vi "new_cursor.vi"(10 "XY":cluster{"X":dbl, "Y":dbl}, 11 "CrsrList":T1(array[cluster])) -> (3 "CrsrList Out":T1(array[cluster]))   [LabVIEW 2023]
panel:
  out "output array":string[](array[string])
  out "Array":bool[](array[boolean])
  out "s? t:f":i32
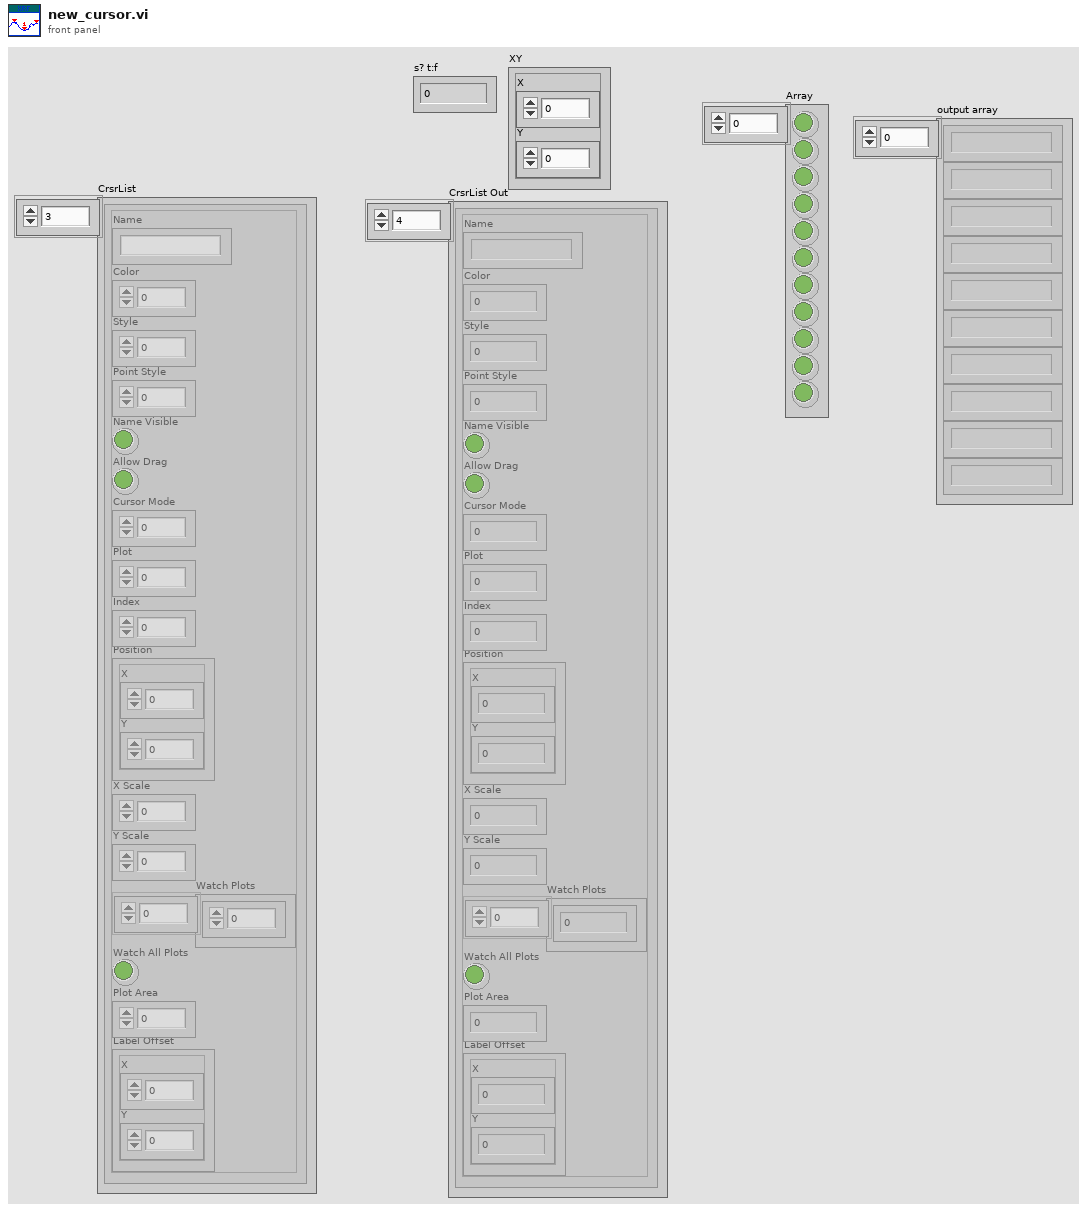
[diagram p1: front panel]
types:
  T1 = cluster{"Name":string, "Color":u32, "Style":i32, "Point Style":i32, "Name Visible":bool, "Allow Drag":bool, "Cursor Mode":u32, "Plot":i32, "Index":i32, "Position":cluster{"X":dbl, "Y":dbl}, "X Scale":u32, "Y Scale":u32, "Watch Plots":i32[], "Watch All Plots":bool, "Plot Area":i32, "Label Offset":cluster{"X":dbl, "Y":dbl}}[]
  T2 = cluster{"Name":string, "Color":u32, "Style":i32, "Point Style":i32, "Name Visible":bool, "Allow Drag":bool, "Cursor Mode":u32, "Plot":i32, "Index":i32, "Position":cluster{"X":dbl, "Y":dbl}, "X Scale":u32, "Y Scale":u32, "Watch Plots":i32[], "Watch All Plots":bool, "Plot Area":i32, "Label Offset":cluster{"X":dbl, "Y":dbl}}
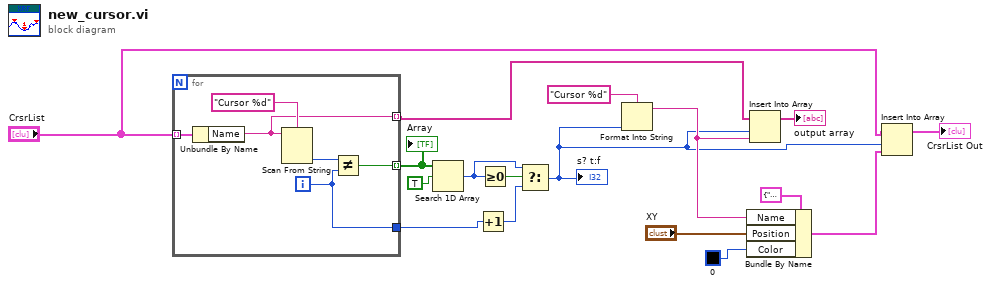
[diagram p0: block diagram]
diagram:
  n1 = for {
    tunnel: "CrsrList" -> [w19] mode=indexing
    tunnel: [w21] -> w16 mode=indexing
    tunnel: [w20] -> w14
    tunnel: [w18] -> w10 mode=indexing
    i -> [w20]
    n2 = Unbundle By Name(w19) -> ("Name"=w18:string)
    n3 = Scan From String(format string="Cursor %d", input string=w18) -> (output 1=w22:i32)  [unwired: 3 in, 3 out]
    n4 = Not Equal?(x=w22, y=w20) -> (x != y?=w21:bool)
  }
  "Array" <- w16
  n5 = Search 1D Array(1D array=w16, element=TRUE) -> (index of element=w12:i32)  [unwired: 1 in]
  n6 = Increment(x=w14) -> (x+1=w13:i32)
  n7 = Greater Or Equal To 0?(x=w12) -> (x >= 0?=w15:bool)
  n8 = Select(t=w12, s=w15, f=w13) -> (s? t:f=w4:i32)
  "s? t:f" <- w4
  n9 = Format Into String(format string="Cursor %d", w4) -> (resulting string=w5:string)  [unwired: 2 in, 1 out]
  n10 = Bundle By Name(cluster=T2 {"Name"="", "Color"=16776704, "Style"=4, "Point Style"=13, "Name Visible"=FALSE, "Allow Drag"=TRUE, "Cursor Mode"=0, "Plot"=0, "Index"=0, "Position"={"X"=0.0, "Y"=0.0}, "X Scale"=0, "Y Scale"=0, "Watch Plots"=[], "Watch All Plots"=FALSE, "Plot Area"=0, "Label Offset"={"X"=0.0, "Y"=0.0}}, "Name"=w5, "Position"="XY", "Color"=u32 0) -> (w3:T2)
  n11 = Insert Into Array(array=w10, index=w4, new element=w5) -> (→"output array":string[])
  n12 = Insert Into Array(array="CrsrList", index=w4, new element=w3) -> (→"CrsrList Out":T1)
